vi "RSZVB Get Calibration Kit.vi"(8 "error in (no error)":errorcluster {"code" format="%.0x"}, 10 "Connector (0: N 50 Ohm)":i32(ring) items=["N 50 Ohm", "N 75 Ohm", "PC 7", "PC 3.5", "2.92 mm", "User 1", "User 2", "SMA"], 11 "VISA session":refnum<visa-resource-name>) -> (0 "error out":errorcluster {"code" format="%.0x"}, 2 "Calibration Kit Name":string, 3 "dup VISA session":refnum<visa-resource-name>)   [LabVIEW 2011]
doc: "This VI queries the calibration kit to be used for a specified connector type.\n\nRemote-control command(s):\n[SENSe<Ch>:]CORRection:CKIT:<conn_type>:SELect?"
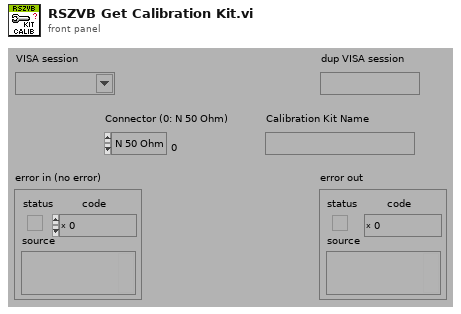
[diagram p1: front panel]
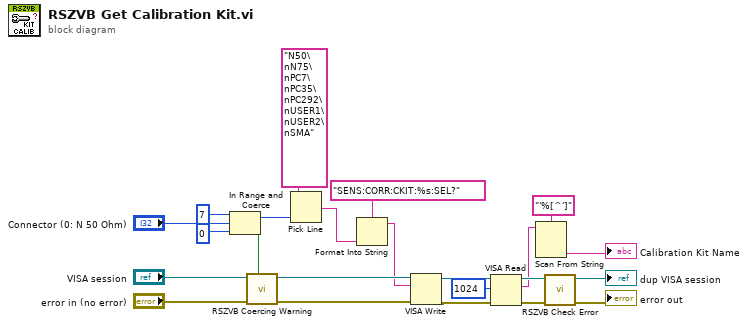
[diagram p0: block diagram]
diagram:
  n1 = In Range and Coerce(upper limit=7 ("lower limit"), x="Connector (0: N 50 Ohm)", lower limit=0) -> (coerced(x)=w17:i32, In Range?=w20:bool)
  n2 = call "RSZVB Coercing Warning.vi"("In Range?"=w20, "error in (no error)"="error in (no error)", "VISA session"="VISA session") -> ("error out"=w22:errorcluster, "dup VISA session"=w23:refnum<visa-resource-name>)  [unwired: 7 in]
  n3 = Pick Line(multi-line string="N50\nN75\nPC7\nPC35\nPC292\nUSER1\nUSER2\nSMA", line index=w17) -> (output string=w15:string)  [unwired: 1 in]
  n4 = Format Into String(format string="SENS:CORR:CKIT:%s:SEL?", w15) -> (resulting string=w14:string)  [unwired: 2 in, 1 out]
  n5 = VISA Write(VISA resource name=w23, write buffer=w14, error in (no error)=w22) -> (VISA resource name out=w5:refnum<visa-resource-name>, error out=w4:errorcluster)  [unwired: 1 out]
  n6 = VISA Read(VISA resource name=w5, byte count=u32 1024 ("byte count (0)"), error in (no error)=w4) -> (VISA resource name out=w10:refnum<visa-resource-name>, read buffer=w2:string, error out=w9:errorcluster)  [unwired: 1 out]
  n7 = Scan From String(format string="'%[^']", input string=w2) -> (output 1=→"Calibration Kit Name":string)  [unwired: 3 in, 3 out]
  n8 = call "RSZVB Check Error.vi"("error in (no error)"=w9, "VISA session"=w10) -> ("error out"=→"error out":errorcluster, "dup VISA session"=→"dup VISA session":refnum<visa-resource-name>)  [unwired: 8 in]
